vi "EnvoiParam (SubVI).vi"(1 "PID 3.3":i8, 2 "PID 3.2":i8, 3 "PID Direction":i8, 4 "PID 2.3":i8, 5 "PID 2.2":i8, 6 "PID Léger":i8, 7 "PID 1.3":i8, 8 "PID 1.2":i8, 9 "PID Fort":i8, 10 "PID vitesse":bool, 11 "ABS":bool) -> (0 "String":string)   [LabVIEW 2013]
panel:
  out "?":bool
  out "?":bool
  out "?":bool
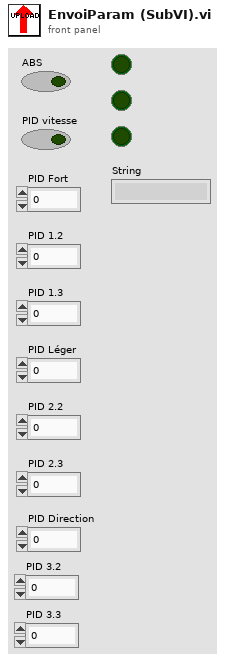
[diagram p1: front panel]
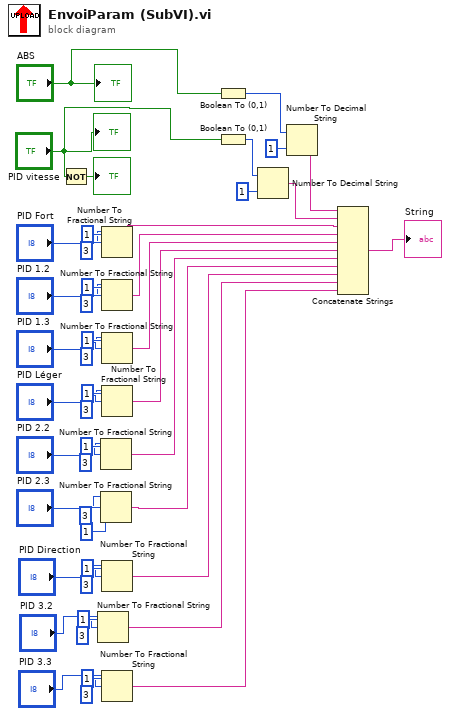
[diagram p0: block diagram]
diagram:
  n1 = Not(x="PID vitesse") -> (.not. x?=→"?":bool)
  n2 = Number To Fractional String(number="PID 3.2", width (-)=i16 3, precision (6)=i16 1) -> (F-format string=w5:string)  [unwired: 1 in]
  n3 = Number To Fractional String(number="PID 2.2", width (-)=i16 3, precision (6)=i16 1) -> (F-format string=w30:string)  [unwired: 1 in]
  n4 = Number To Fractional String(number="PID 2.3", width (-)=i16 3, precision (6)=i16 1) -> (F-format string=w31:string)  [unwired: 1 in]
  n5 = Number To Fractional String(number="PID Fort", width (-)=i16 3, precision (6)=i16 1) -> (F-format string=w26:string)  [unwired: 1 in]
  n6 = Number To Fractional String(number="PID 1.2", width (-)=i16 3, precision (6)=i16 1) -> (F-format string=w27:string)  [unwired: 1 in]
  n7 = Number To Fractional String(number="PID 1.3", width (-)=i16 3, precision (6)=i16 1) -> (F-format string=w28:string)  [unwired: 1 in]
  n8 = Number To Fractional String(number="PID Léger", width (-)=i16 3, precision (6)=i16 1) -> (F-format string=w29:string)  [unwired: 1 in]
  n9 = Number To Fractional String(number="PID Direction", width (-)=i16 3, precision (6)=i16 1) -> (F-format string=w6:string)  [unwired: 1 in]
  n10 = Number To Fractional String(number="PID 3.3", width (-)=i16 3, precision (6)=i16 1) -> (F-format string=w4:string)  [unwired: 1 in]
  n11 = Boolean To (0,1)(Boolean="ABS") -> (0, 1=w25:i16)
  n12 = Boolean To (0,1)(Boolean="PID vitesse") -> (0, 1=w24:i16)
  n13 = Number To Decimal String(number=w24, width (-)=i16 1) -> (decimal integer string=w23:string)
  n14 = Number To Decimal String(number=w25, width (-)=i16 1) -> (decimal integer string=w16:string)
  n15 = Concatenate Strings(w16, w23, w26, w27, w28, w29, w30, w31, w6, w5, w4) -> (→"String":string)
  "?" <- "ABS"
  "?" <- "PID vitesse"
